vi "Protect File.vi"(0 "VISA resource name":refnum<visa-resource-name>, 5 "Protection Mode (0:Hard Copy)":i32(ring) items=["Hard Copy", "Parameter", "System Info", "Trace"], 7 "Application (0:Spectrum Analyzer)":i32(ring) items=["Spectrum Analyzer", "Phase Noise"], 9 "Protect Filename (TEST)":string="TEST", 11 "error in (no error)":errorcluster, 12 "Driver Letter (D)":string="D", 13 "Protection (1:On)":i32(ring)=1 items=["Off", "On"]) -> (4 "VISA resource name out":refnum<visa-resource-name>, 15 "error out":errorcluster)   [LabVIEW 2020, in "Anritsu Signal Analyzer Series.lvlib"]
doc: "Protects a screen hardcopy file saved in the internal hard disk to the specified device.\nProtects a parameter file saved in the internal hard disk to the specified device.\nProtects a system information file saved in the internal hard disk to the specified device.\nProtects a trace file saved in the internal hard disk to the specified device."
uses:
  Anritsu Signal Analyzer Series.lvlib
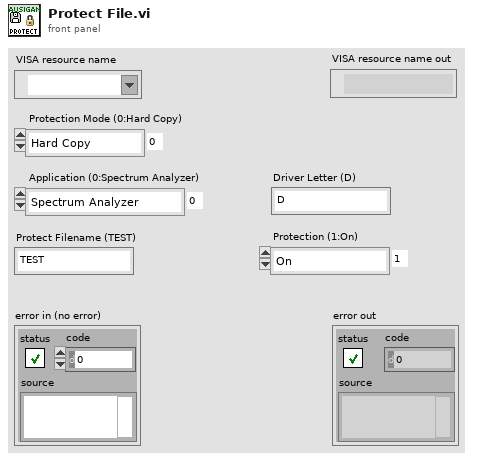
[diagram p1: front panel]
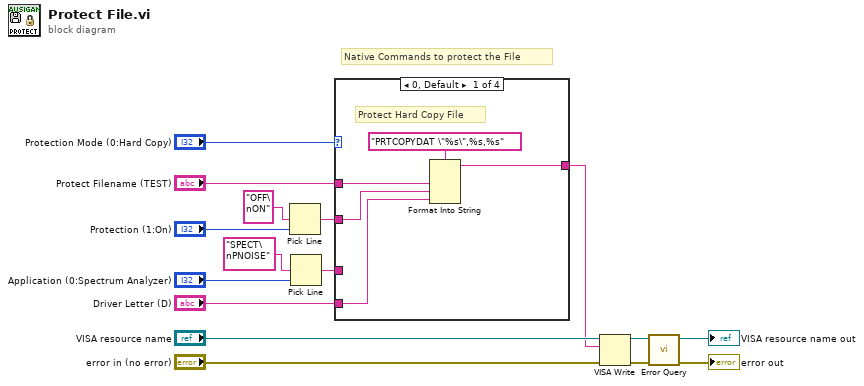
[diagram p0: block diagram]
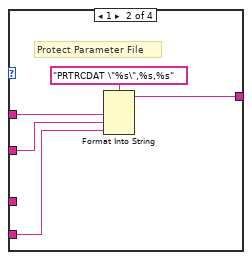
[diagram p2: hidden frame]
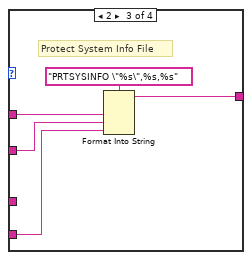
[diagram p3: hidden frame]
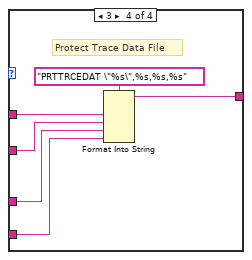
[diagram p4: hidden frame]
diagram:
  # "Native Commands to protect the File"
  n1 = Pick Line(multi-line string="OFF\nON" ("_Case1"), line index="Protection (1:On)") -> (output string=w6:string)  [unwired: 1 in]
  n2 = Pick Line(multi-line string="SPECT\nPNOISE", line index="Application (0:Spectrum Analyzer)") -> (output string=w3:string)  [unwired: 1 in]
  n3 = case shown="0, Default" "Protection Mode (0:Hard Copy)" {
    tunnel: "Protect Filename (TEST)" -> [w21 w26 w31 w37]
    tunnel: "Driver Letter (D)" -> [w19 w24 w29 w33]
    tunnel: w6 -> [w20 w25 w30 w36]
    tunnel: w3 -> [_ _ _ w32]
    tunnel: [w17 w22 w27 w34] -> w7
    frame 0, Default {
      # "Protect Hard Copy File"
      n4 = Format Into String(format string="PRTCOPYDAT \"%s\",%s,%s" ("_CommandSet"), w21, w20, w19) -> (resulting string=w17:string)  [unwired: 2 in, 1 out]
    }
    frame 1 {
      # "Protect Parameter File"
      n5 = Format Into String(format string="PRTRCDAT \"%s\",%s,%s" ("_CommandSet"), w26, w25, w24) -> (resulting string=w22:string)  [unwired: 2 in, 1 out]
    }
    frame 2 {
      # "Protect System Info File"
      n6 = Format Into String(format string="PRTSYSINFO \"%s\",%s,%s" ("_CommandSet"), w31, w30, w29) -> (resulting string=w27:string)  [unwired: 2 in, 1 out]
    }
    frame 3 {
      # "Protect Trace Data File"
      n7 = Format Into String(format string="PRTTRCEDAT \"%s\",%s,%s,%s" ("_CommandSet"), w37, w36, w32, w33) -> (resulting string=w34:string)  [unwired: 2 in, 1 out]
    }
  }
  n8 = VISA Write(VISA resource name="VISA resource name", write buffer=w7, error in (no error)="error in (no error)") -> (VISA resource name out=w8:refnum<visa-resource-name>, error out=w9:errorcluster)  [unwired: 1 out]
  n9 = call "Error Query.vi"("error in (no error)"=w9, "VISA resource name"=w8) -> ("error out"=→"error out":errorcluster, "VISA resource name out"=→"VISA resource name out":refnum<visa-resource-name>)  [unwired: 6 in, 2 out]
